vi "inout logic (SubVI).vi"(8 "Sensor 2 (T-2)":bool, 9 "Sensor 2 (T-1)":bool, 10 "Sensor 1 (T-2)":bool, 11 "Sensor 1 (T-1)":bool) -> (2 "IN":bool, 3 "OUT":bool)   [LabVIEW 2022 SP3]
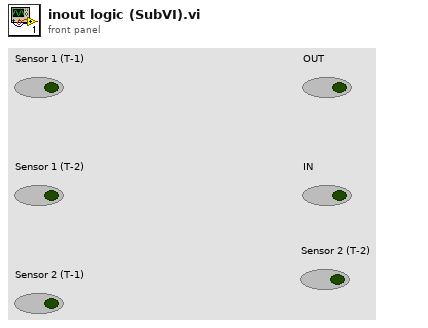
[diagram p1: front panel]
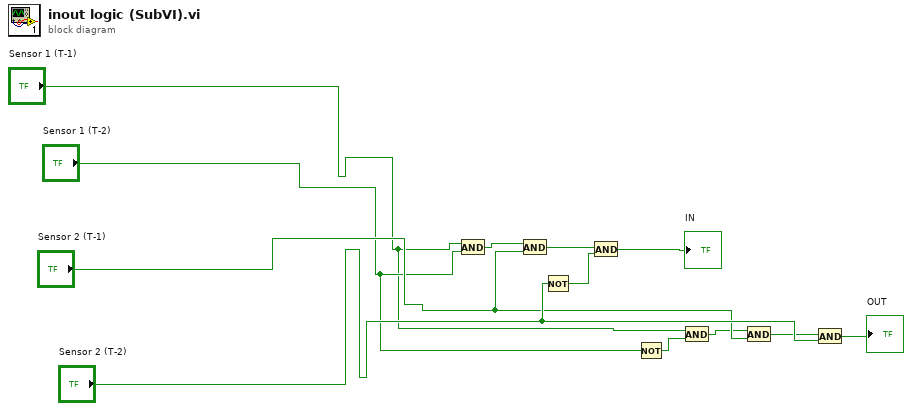
[diagram p0: block diagram]
diagram:
  n1 = And(x="Sensor 1 (T-1)", y="Sensor 1 (T-2)") -> (x .and. y?=w1:bool)
  n2 = And(x=w1, y="Sensor 2 (T-1)") -> (x .and. y?=w2:bool)
  n3 = Not(x="Sensor 2 (T-2)") -> (.not. x?=w3:bool)
  n4 = And(x=w2, y=w3) -> (x .and. y?=→"IN":bool)
  n5 = Not(x="Sensor 1 (T-2)") -> (.not. x?=w6:bool)
  n6 = And(x="Sensor 1 (T-1)", y=w6) -> (x .and. y?=w4:bool)
  n7 = And(x=w4, y="Sensor 2 (T-1)") -> (x .and. y?=w5:bool)
  n8 = And(x=w5, y="Sensor 2 (T-2)") -> (x .and. y?=→"OUT":bool)
